vi "MoveElevatorDown.vi"(8 "error in (no error)":errorcluster) -> (0 "error out":errorcluster)   [LabVIEW 2017, in "Thermal Shock.lvlib"]
uses:
  Thermal Shock.lvlib
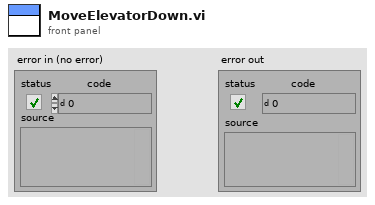
[diagram p1: front panel]
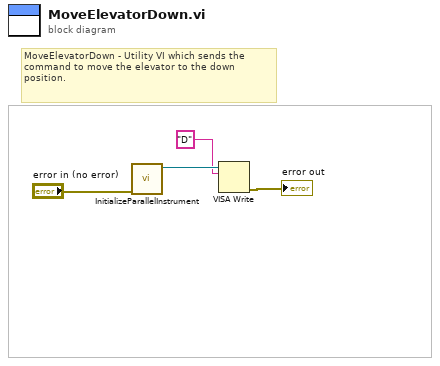
[diagram p0: block diagram]
diagram:
  # "MoveElevatorDown - Utility VI which sends the command to move the elevator to the down position."
  n1 = call "InitializeParallelInstrument.vi"("error in (no error)"="error in (no error)") -> ("Parallel Instrument OUT"=w3:refnum<visa-resource-name>)  [unwired: 9 in, 1 out]
  n2 = VISA Write(VISA resource name=w3, write buffer="D") -> (error out=→"error out":errorcluster)  [unwired: 1 in, 2 out]
